vi "OAT Polar Plot Indicator.vi"() -> ()   [LabVIEW 2017]
doc: "Uses the Polar Plot to display the order magnitude and phase on a customized picture control."
uses:
  <vilib>/addons/Sound and Vibration/Order Analysis/Backward Compatibility/OAT Polar Plot (Auto Label).vi
panel:
  out "Polar Plot":picture
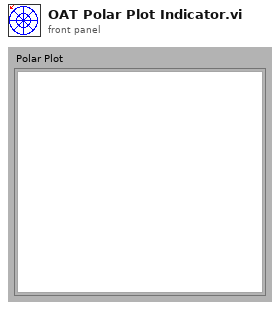
[diagram p1: front panel]
types:
  T1 = typedef "LVBoundsTypeDef.ctl" = cluster{"Width":u32, "Height":u32}
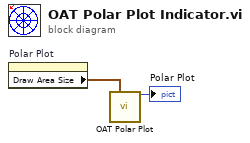
[diagram p0: block diagram]
diagram:
  n1 = property on="Polar Plot" class="Pict"() -> ("Draw Area Size"=w2:T1)  [unwired: 2 in, 2 out]
  n2 = call-poly <vilib>:"OAT Polar Plot.vi"("picture\ndimensions (w,h)"=w2) -> ("new picture"=→"Polar Plot":picture)  [unwired: 13 in, 1 out]
